vi "Main.vi"() -> ()   [LabVIEW 2013]
uses:
  <vilib>/Utility/error.llb/DialogType.ctl
panel:
  in  "Выкл2":bool
  in  "Выкл":bool
  out "K2 conn":bool caption="NC"
  out "K1 conn":bool caption="NC"
  in  "IP 2":string="172.16.21.127"
  in  "IP 1":string="172.16.21.126"
  in  "А 2":dbl min=0.0 max=30.0 step=0.001 format="%.3f"
  in  "NeedToSetCurrent 2":bool
  out "V 3":string
  out "А 3":string
  in  "Вкл2":bool
  out "Out":bool
  in  "V 2":dbl min=0.0 max=30.0 step=0.1 format="%.1f"
  in  "NeedToSetVoltage 2":bool
  out "message 2":string=" INSTRUCTIONS:\r\rNormal Use:  When using subVIs that incorporate the error in/error out (or error I/O) structure, place this handler where you want to inform the user of an error, typically at the end of the I/O data path, as the last action of the program.  If the error in error? is ERROR, the handler creates a message describing the error and its source.  If the type of dialog = 1 (default), the message is displayed to the user, who can only acknowedge it.  If the type = 2, the user can acknowledge the message or abort execution; aborting a program with active I/O is not recommended.  If the type = 0, no message is displayed; this is used to process the error programmatically, and the error out cluster elements are wired to individual terminals for that reason.  \r\rOther Use:\n\r\nlocal testing.  To test the error code of a subVI or function that does not have the error I/O structure, you can wire its error code and a source string to the local error code and error source inputs.  If error in error? indicates no error and error code is not equal to 0, the local code and source are substituted for the error in values, and error? is set TRUE (ERROR)."
  out "conn src 2":refnum<k5>
  out "conn src":refnum<k5>
  in  "stop":bool
  out "message":string=" INSTRUCTIONS:\r\rNormal Use:  When using subVIs that incorporate the error in/error out (or error I/O) structure, place this handler where you want to inform the user of an error, typically at the end of the I/O data path, as the last action of the program.  If the error in error? is ERROR, the handler creates a message describing the error and its source.  If the type of dialog = 1 (default), the message is displayed to the user, who can only acknowedge it.  If the type = 2, the user can acknowledge the message or abort execution; aborting a program with active I/O is not recommended.  If the type = 0, no message is displayed; this is used to process the error programmatically, and the error out cluster elements are wired to individual terminals for that reason.  \r\rOther Use:\n\r\nlocal testing.  To test the error code of a subVI or function that does not have the error I/O structure, you can wire its error code and a source string to the local error code and error source inputs.  If error in error? indicates no error and error code is not equal to 0, the local code and source are substituted for the error in values, and error? is set TRUE (ERROR)."
  in  "V":dbl min=0.0 max=30.0 step=0.1 format="%.1f"
  in  "А":dbl min=0.0 max=72.0 step=0.001 format="%.3f"
  in  "NeedToSetVoltage":bool
  in  "NeedToSetCurrent":bool
  out "V":string
  out "А":string
  in  "Вкл.":bool
  out "Out":bool
  # "LEBT HILAC corrector supply"
  # "Settings"
  # "Settings"
  # "Horizontal corrector voltage"
  # "Vertical corrector voltage"
  # "Horizontal"
  # "Vertical"
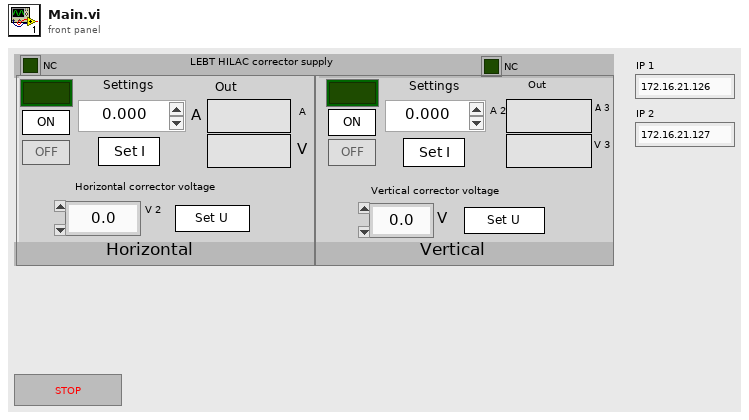
[diagram p1: front panel]
types:
  T1 = enum8{"Enabled", "Disabled", "Disabled and Grayed Out"}
  T2 = typedef "DialogType.ctl" = u16
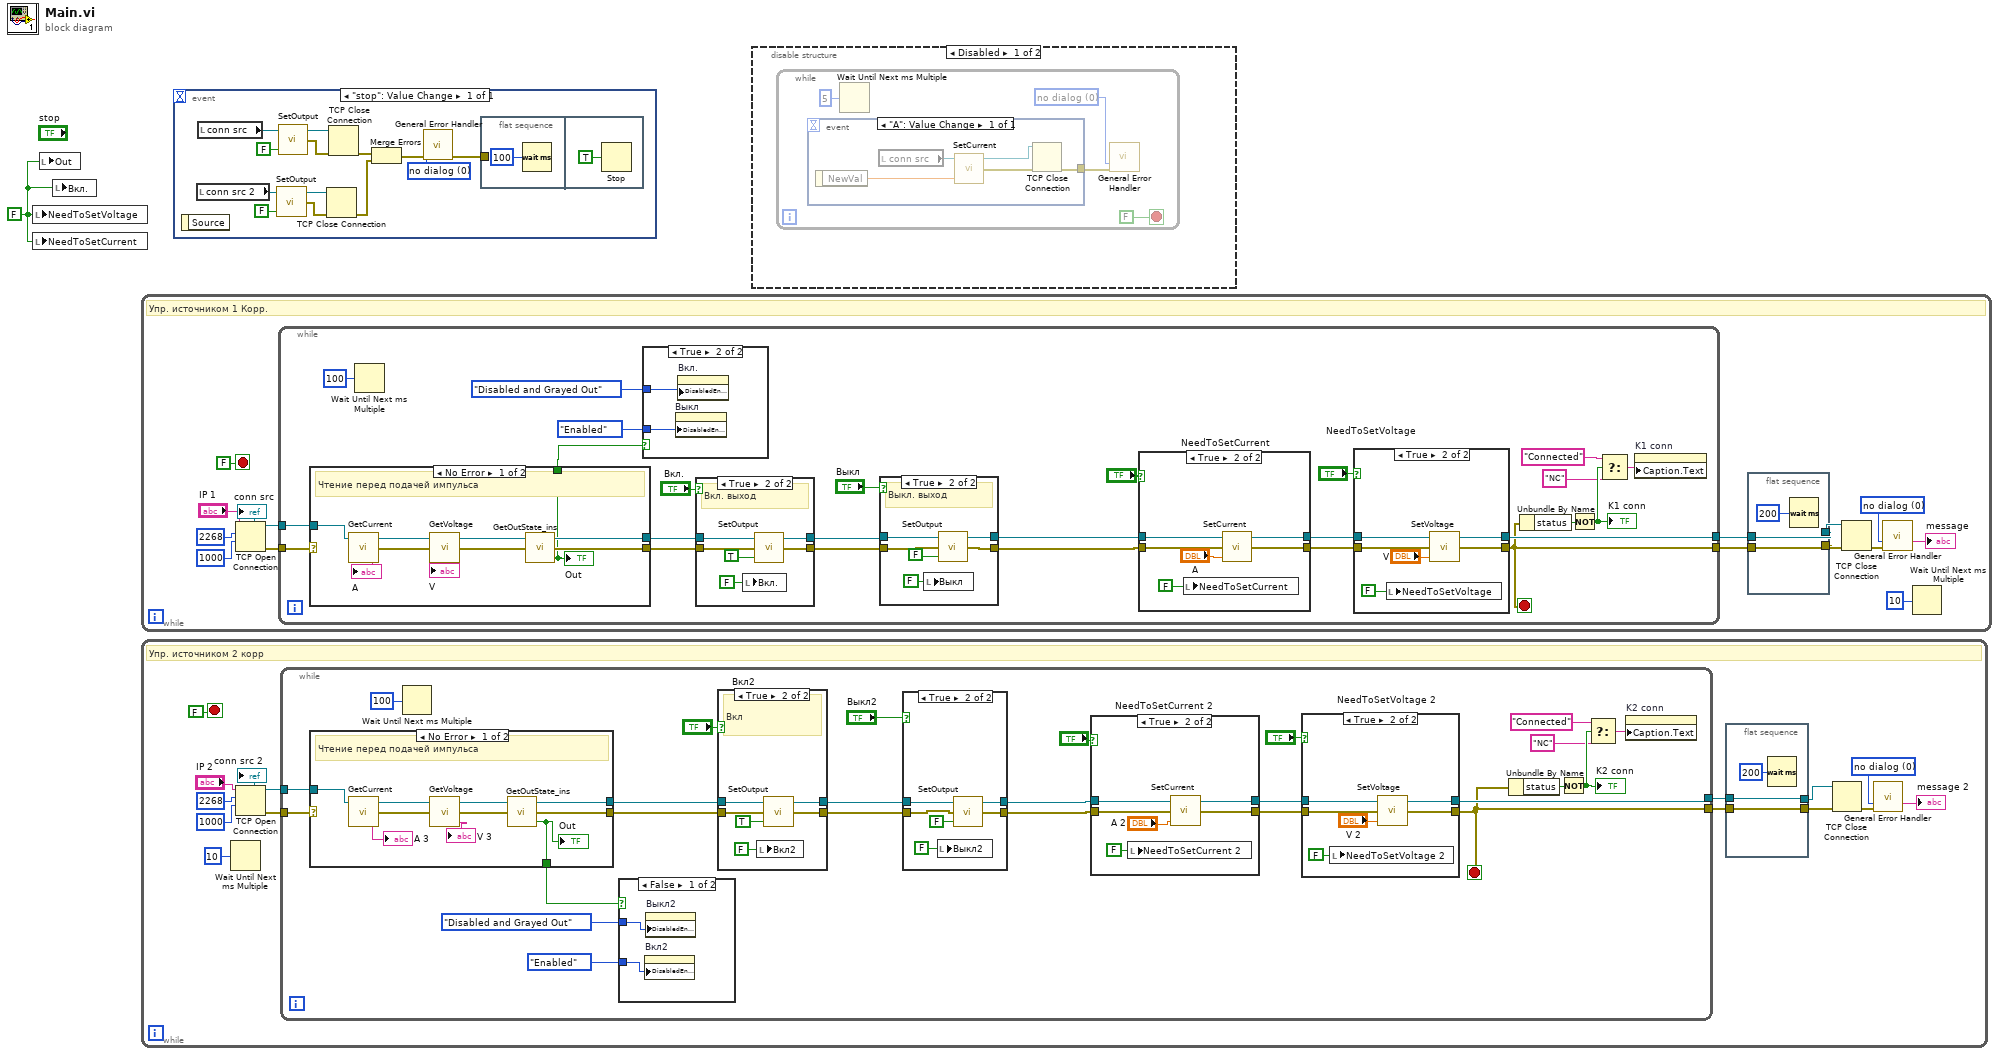
[diagram p0: block diagram]
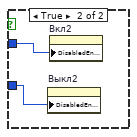
[diagram p4: hidden frame]
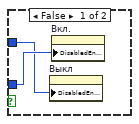
[diagram p10: hidden frame]
diagram:
  w1 = FALSE ("Connect")
  n1 = local write "NeedToSetVoltage"(w1) -> ()
  n2 = local write "NeedToSetCurrent"(w1) -> ()
  n3 = local write "Out"(w1) -> ()
  n4 = local write "Вкл."(w1) -> ()
  n5 = while {
    stop <- FALSE stop-if-true
    w10 = T2 0 items=["no dialog", "OK message", "continue or stop message", "OK message + warnings", "continue/stop + warnings"] ("type of dialog (OK msg:1)")
    # "Упр. источником 1 Корр."
    n6 = TCP Open Connection(address="IP 1", remote port or service name=u16 2268 ("Port"), timeout ms (60000)=1000) -> (connection ID=w12:refnum<k5>, error out=w13:errorcluster)  [unwired: 1 in, 1 out]
    "conn src" <- w12
    n7 = while {
      tunnel: w13 -> [w43]
      tunnel: w12 -> [w42]
      tunnel: [w41] -> w5
      tunnel: [w32] -> w4
      stop <- w32 stop-if-true
      n8 = case shown="No Error" w43 {
        selector: w43 -> [_ w82]
        tunnel: w42 -> [w77 w83]
        tunnel: [w73 w82] -> w37
        tunnel: [w74 w83] -> w36
        tunnel: [w72 _] -> w26
        frame No Error {
          # "Чтение перед подачей импульса"
          n9 = call "GetCurrent.vi"("connection ID"=w77) -> ("Current"=→"А":string, "error out"=w78:errorcluster, "connection ID out"=w80:refnum<k5>)  [unwired: 1 in, 1 out]
          n10 = call "GetVoltage.vi"("error in"=w78, "connection ID"=w80) -> ("Voltage"=→"V":string, "error out"=w76:errorcluster, "connection ID out"=w75:refnum<k5>)  [unwired: 1 out]
          n11 = call "GetOutState_ins.vi"("error in"=w76, "connection ID"=w75) -> ("OutState"=w72:bool, "error out"=w73:errorcluster, "connection ID out"=w74:refnum<k5>)  [unwired: 1 out]
          "Out" <- w72
        }
        frame Error {
        }
      }
      n12 = Wait Until Next ms Multiple(millisecond multiple=u32 100) -> ()  [unwired: 1 out]
      n13 = case shown="True" w26 {
        tunnel: T1."Enabled" ("Disabled") -> [w53 w55]
        tunnel: T1."Disabled and Grayed Out" ("Disabled") -> [w52 w54]
        frame False {
          n14 = property on="Выкл" class="Bool (strict)"("DisabledEnum"=w52) -> ()  [unwired: 2 in, 2 out]
          n15 = property on="Вкл." class="Bool (strict)"("DisabledEnum"=w53) -> ()  [unwired: 2 in, 2 out]
        }
        frame True {
          n16 = property on="Выкл" class="Bool (strict)"("DisabledEnum"=w55) -> ()  [unwired: 2 in, 2 out]
          n17 = property on="Вкл." class="Bool (strict)"("DisabledEnum"=w54) -> ()  [unwired: 2 in, 2 out]
        }
      }
      n18 = case shown="True" "Вкл." {
        tunnel: w37 -> [w64 w71]
        tunnel: w36 -> [w65 w70]
        tunnel: [w65 w69] -> w22
        tunnel: [w64 w68] -> w21
        frame False {
          # "Ручное управление выходом"
        }
        frame True {
          # "Вкл. выход"
          n19 = local write "Вкл."(FALSE ("Вкл.")) -> ()
          n20 = call "SetOutput.vi"("State"=TRUE, "error in"=w71, "connection ID"=w70) -> ("error out"=w68:errorcluster, "connection ID out"=w69:refnum<k5>)  [unwired: 1 out]
        }
      }
      n21 = case shown="True" "Выкл" {
        tunnel: w21 -> [w44 w51]
        tunnel: w22 -> [w45 w50]
        tunnel: [w45 w49] -> w20
        tunnel: [w44 w48] -> w19
        frame False {
          # "Ручное управление выходом"
        }
        frame True {
          # "Выкл. выход"
          n22 = local write "Выкл"(FALSE ("Вкл.")) -> ()
          n23 = call "SetOutput.vi"("State"=FALSE, "error in"=w51, "connection ID"=w50) -> ("error out"=w48:errorcluster, "connection ID out"=w49:refnum<k5>)  [unwired: 1 out]
        }
      }
      n24 = case shown="True" "NeedToSetCurrent" {
        tunnel: [w57 w62] -> w40
        tunnel: [w56 w60] -> w38
        tunnel: w20 -> [w57 w59]
        tunnel: w19 -> [w56 w58]
        frame False {
        }
        frame True {
          n25 = local write "NeedToSetCurrent"(FALSE ("NeedToSetOutput")) -> ()
          n26 = call "SetCurrent.vi"("Current"="А", "error in"=w58, "connection ID"=w59) -> ("error out"=w60:errorcluster, "connection ID out"=w62:refnum<k5>)  [unwired: 1 out]
        }
      }
      n27 = case shown="True" "NeedToSetVoltage" {
        tunnel: w40 -> [w85 w91]
        tunnel: [w85 w88] -> w41
        tunnel: w38 -> [w84 w87]
        tunnel: [w84 w86] -> w32
        frame False {
        }
        frame True {
          n28 = local write "NeedToSetVoltage"(FALSE ("NeedToSetOutput")) -> ()
          n29 = call "SetVoltage.vi"("Voltage"="V", "error in"=w87, "connection ID"=w91) -> ("error out"=w86:errorcluster, "connection ID out"=w88:refnum<k5>)  [unwired: 1 out]
        }
      }
      n30 = Unbundle By Name(w32) -> ("status"=w31:bool)
      n31 = Not(x=w31) -> (.not. x?=w30:bool)
      "K1 conn" <- w30
      n32 = Select(t="Connected", s=w30, f="NC") -> (s? t:f=w29:string)
      n33 = property on="K1 conn" class="Bool (strict)"("Caption.Text"=w29) -> ()  [unwired: 2 in, 2 out]
    }
    n34 = flat-sequence {
      tunnel: [w18] -> w6
      tunnel: w5 -> [w18]
      tunnel: [w17] -> w3
      tunnel: w4 -> [w17]
      frame #0 {
        n35 = Wait (ms)(milliseconds to wait=u32 200 ("millisecond multiple")) -> ()  [unwired: 1 out]
      }
    }
    n36 = TCP Close Connection(connection ID=w6, error in (no error)=w3) -> (error out=w11:errorcluster)  [unwired: 2 out]
    n37 = call <vilib>:"General Error Handler.vi"("type of dialog (OK msg:1)"=w10, "error in (no error)"=w11) -> ("message"=→"message":string)  [unwired: 9 in, 4 out]
    n38 = Wait Until Next ms Multiple(millisecond multiple=u32 10) -> ()  [unwired: 1 out]
  }
  n39 = while {
    stop <- FALSE stop-if-true
    w100 = T2 0 items=["no dialog", "OK message", "continue or stop message", "OK message + warnings", "continue/stop + warnings"] ("type of dialog (OK msg:1)")
    # "Упр. источником 2 корр"
    n40 = Wait Until Next ms Multiple(millisecond multiple=u32 10 ("milliseconds to wait")) -> ()  [unwired: 1 out]
    n41 = TCP Open Connection(address="IP 2", remote port or service name=u16 2268 ("Port"), timeout ms (60000)=1000) -> (connection ID=w102:refnum<k5>, error out=w103:errorcluster)  [unwired: 1 in, 1 out]
    "conn src 2" <- w102
    n42 = while {
      tunnel: w103 -> [w133]
      tunnel: w102 -> [w132]
      tunnel: [w131] -> w95
      tunnel: [w117] -> w93
      stop <- w117 stop-if-true
      n43 = case shown="No Error" w133 {
        selector: w133 -> [_ w164]
        tunnel: w132 -> [w161 w165]
        tunnel: [w156 w164] -> w127
        tunnel: [w155 w165] -> w126
        tunnel: [w154 _] -> w114
        frame No Error {
          # "Чтение перед подачей импульса"
          n44 = call "GetCurrent.vi"("connection ID"=w161) -> ("Current"=→"А 3":string, "error out"=w162:errorcluster, "connection ID out"=w163:refnum<k5>)  [unwired: 1 in, 1 out]
          n45 = call "GetVoltage.vi"("error in"=w162, "connection ID"=w163) -> ("Voltage"=→"V 3":string, "error out"=w157:errorcluster, "connection ID out"=w158:refnum<k5>)  [unwired: 1 out]
          n46 = call "GetOutState_ins.vi"("error in"=w157, "connection ID"=w158) -> ("OutState"=w154:bool, "error out"=w156:errorcluster, "connection ID out"=w155:refnum<k5>)  [unwired: 1 out]
          "Out" <- w154
        }
        frame Error {
        }
      }
      n47 = Wait Until Next ms Multiple(millisecond multiple=u32 100) -> ()  [unwired: 1 out]
      n48 = case shown="False" w114 {
        tunnel: T1."Disabled and Grayed Out" ("Disabled") -> [w142 w145]
        tunnel: T1."Enabled" ("Disabled") -> [w143 w144]
        frame False {
          n49 = property on="Вкл2" class="Bool (strict)"("DisabledEnum"=w143) -> ()  [unwired: 2 in, 2 out]
          n50 = property on="Выкл2" class="Bool (strict)"("DisabledEnum"=w142) -> ()  [unwired: 2 in, 2 out]
        }
        frame True {
          n51 = property on="Выкл2" class="Bool (strict)"("DisabledEnum"=w144) -> ()  [unwired: 2 in, 2 out]
          n52 = property on="Вкл2" class="Bool (strict)"("DisabledEnum"=w145) -> ()  [unwired: 2 in, 2 out]
        }
      }
      n53 = case shown="True" "Вкл2" {
        tunnel: w127 -> [w146 w153]
        tunnel: w126 -> [w147 w152]
        tunnel: [w147 w151] -> w112
        tunnel: [w146 w150] -> w111
        frame False {
          # "Вкл."
        }
        frame True {
          # "Вкл"
          n54 = local write "Вкл2"(FALSE ("Вкл2")) -> ()
          n55 = call "SetOutput.vi"("State"=TRUE, "error in"=w153, "connection ID"=w152) -> ("error out"=w150:errorcluster, "connection ID out"=w151:refnum<k5>)  [unwired: 1 out]
        }
      }
      n56 = case shown="True" "Выкл2" {
        tunnel: w112 -> [w135 w140]
        tunnel: w111 -> [w134 w139]
        tunnel: [w135 w138] -> w110
        tunnel: [w134 w137] -> w109
        frame False {
        }
        frame True {
          n57 = local write "Выкл2"(FALSE ("Выкл2")) -> ()
          n58 = call "SetOutput.vi"("State"=FALSE, "error in"=w139, "connection ID"=w140) -> ("error out"=w137:errorcluster, "connection ID out"=w138:refnum<k5>)  [unwired: 1 out]
        }
      }
      n59 = case shown="True" "NeedToSetCurrent 2" {
        tunnel: [w175 w181] -> w130
        tunnel: [w174 w179] -> w128
        tunnel: w110 -> [w175 w178]
        tunnel: w109 -> [w174 w177]
        frame False {
        }
        frame True {
          n60 = local write "NeedToSetCurrent 2"(FALSE ("NeedToSetOutput")) -> ()
          n61 = call "SetCurrent.vi"("Current"="А 2", "error in"=w177, "connection ID"=w178) -> ("error out"=w179:errorcluster, "connection ID out"=w181:refnum<k5>)  [unwired: 1 out]
        }
      }
      n62 = case shown="True" "NeedToSetVoltage 2" {
        tunnel: w130 -> [w167 w173]
        tunnel: [w167 w170] -> w131
        tunnel: w128 -> [w166 w169]
        tunnel: [w166 w168] -> w117
        frame False {
        }
        frame True {
          n63 = local write "NeedToSetVoltage 2"(FALSE ("NeedToSetOutput")) -> ()
          n64 = call "SetVoltage.vi"("Voltage"="V 2", "error in"=w169, "connection ID"=w173) -> ("error out"=w168:errorcluster, "connection ID out"=w170:refnum<k5>)  [unwired: 1 out]
        }
      }
      n65 = Unbundle By Name(w117) -> ("status"=w122:bool)
      n66 = Not(x=w122) -> (.not. x?=w121:bool)
      "K2 conn" <- w121
      n67 = Select(t="Connected", s=w121, f="NC") -> (s? t:f=w120:string)
      n68 = property on="K2 conn" class="Bool (strict)"("Caption.Text"=w120) -> ()  [unwired: 2 in, 2 out]
    }
    n69 = flat-sequence {
      tunnel: [w108] -> w94
      tunnel: w95 -> [w108]
      tunnel: w93 -> [w107]
      tunnel: [w107] -> w92
      frame #0 {
        n70 = Wait (ms)(milliseconds to wait=u32 200 ("millisecond multiple")) -> ()  [unwired: 1 out]
      }
    }
    n71 = TCP Close Connection(connection ID=w94, error in (no error)=w92) -> (error out=w101:errorcluster)  [unwired: 2 out]
    n72 = call <vilib>:"General Error Handler.vi"("type of dialog (OK msg:1)"=w100, "error in (no error)"=w101) -> ("message"=→"message 2":string)  [unwired: 9 in, 4 out]
  }
  n73 = event shown="[0] \"stop\": Value Change" {
    selector: _ -> [_]
    dyn-events: _ -> [_]
    timeout: _ -> [_]
    event "stop": Value Change {
      w192 = T2 0 items=["no dialog", "OK message", "continue or stop message", "OK message + warnings", "continue/stop + warnings"] ("type of dialog (OK msg:1)")
      n74 = event-data() -> ()  [unwired: 1 in, 1 out]
      n75 = local read "conn src 2"() -> (w183:refnum<k5>)
      n76 = local read "conn src"() -> (w190:refnum<k5>)
      n77 = call "SetOutput.vi"("State"=FALSE, "connection ID"=w183) -> ("error out"=w185:errorcluster, "connection ID out"=w184:refnum<k5>)  [unwired: 1 in, 1 out]
      n78 = call "SetOutput.vi"("State"=FALSE, "connection ID"=w190) -> ("error out"=w188:errorcluster, "connection ID out"=w189:refnum<k5>)  [unwired: 1 in, 1 out]
      n79 = TCP Close Connection(connection ID=w184, error in (no error)=w185) -> (error out=w182:errorcluster)  [unwired: 1 in, 1 out]
      n80 = TCP Close Connection(connection ID=w189, error in (no error)=w188) -> (error out=w194:errorcluster)  [unwired: 1 in, 1 out]
      n81 = Merge Errors(w194, w182) -> (w193:errorcluster)
      n82 = call <vilib>:"General Error Handler.vi"("type of dialog (OK msg:1)"=w192, "error in (no error)"=w193) -> ("error out"=w191:errorcluster)  [unwired: 9 in, 4 out]
      n83 = flat-sequence {
        tunnel: w191 -> [_]
        frame #0 {
          n84 = Wait (ms)(milliseconds to wait=u32 100) -> ()  [unwired: 1 out]
        }
        frame #1 {
          n85 = Stop(stop? (T)=TRUE) -> ()
        }
      }
    }
  }
  n86 = disable-structure shown="Disabled" {
    frame Disabled {
      n87 = while {
        stop <- FALSE stop-if-true
        w200 = T2 0 items=["no dialog", "OK message", "continue or stop message", "OK message + warnings", "continue/stop + warnings"] ("type of dialog (OK msg:1)")
        n88 = event shown="[0] \"А\": Value Change" {
          selector: _ -> [_]
          dyn-events: _ -> [_]
          timeout: _ -> [_]
          tunnel: [w201] -> w199
          event "А": Value Change {
            n89 = event-data() -> ("NewVal"=w205:dbl)  [unwired: 1 in]
            n90 = local read "conn src"() -> (w204:refnum<k5>)
            n91 = call "SetCurrent.vi"("Current"=w205, "connection ID"=w204) -> ("error out"=w202:errorcluster, "connection ID out"=w203:refnum<k5>)  [unwired: 1 in, 1 out]
            n92 = TCP Close Connection(connection ID=w203, error in (no error)=w202) -> (error out=w201:errorcluster)  [unwired: 2 out]
          }
        }
        n93 = Wait Until Next ms Multiple(millisecond multiple=u32 5) -> ()  [unwired: 1 out]
        n94 = call <vilib>:"General Error Handler.vi"("type of dialog (OK msg:1)"=w200, "error in (no error)"=w199) -> ()  [unwired: 9 in, 5 out]
      }
    }
    frame Enabled {
    }
  }
